vi "gyro_get_statistics.vi"(8 "error in":errorcluster, 11 "all in one package in":T1 {"time informations"."length" format="%<%H:%M:%S%3u>t"; "actigraph settings"."id" format="%02d"; "actigraph settings"."range code" format="%02x"; "actigraph settings"."rate code" format="%02x"}) -> (0 "error out":errorcluster, 3 "all in one package out":T1 {"time informations"."length" format="%<%H:%M:%S%3u>t"; "actigraph settings"."id" format="%02d"; "actigraph settings"."range code" format="%02x"; "actigraph settings"."rate code" format="%02x"})   [LabVIEW 2019]
uses:
  <vilib>/Analysis/NI_AALBase.lvlib
  Controls/gyro_control_memory_structure.ctl
  Controls/gyro_control_measurement_settings.ctl
  Controls/gyro_control_time_informations.ctl
  Controls/gyro_control_measurement_data.ctl
  Controls/gyro_control_all_in_one_package.ctl
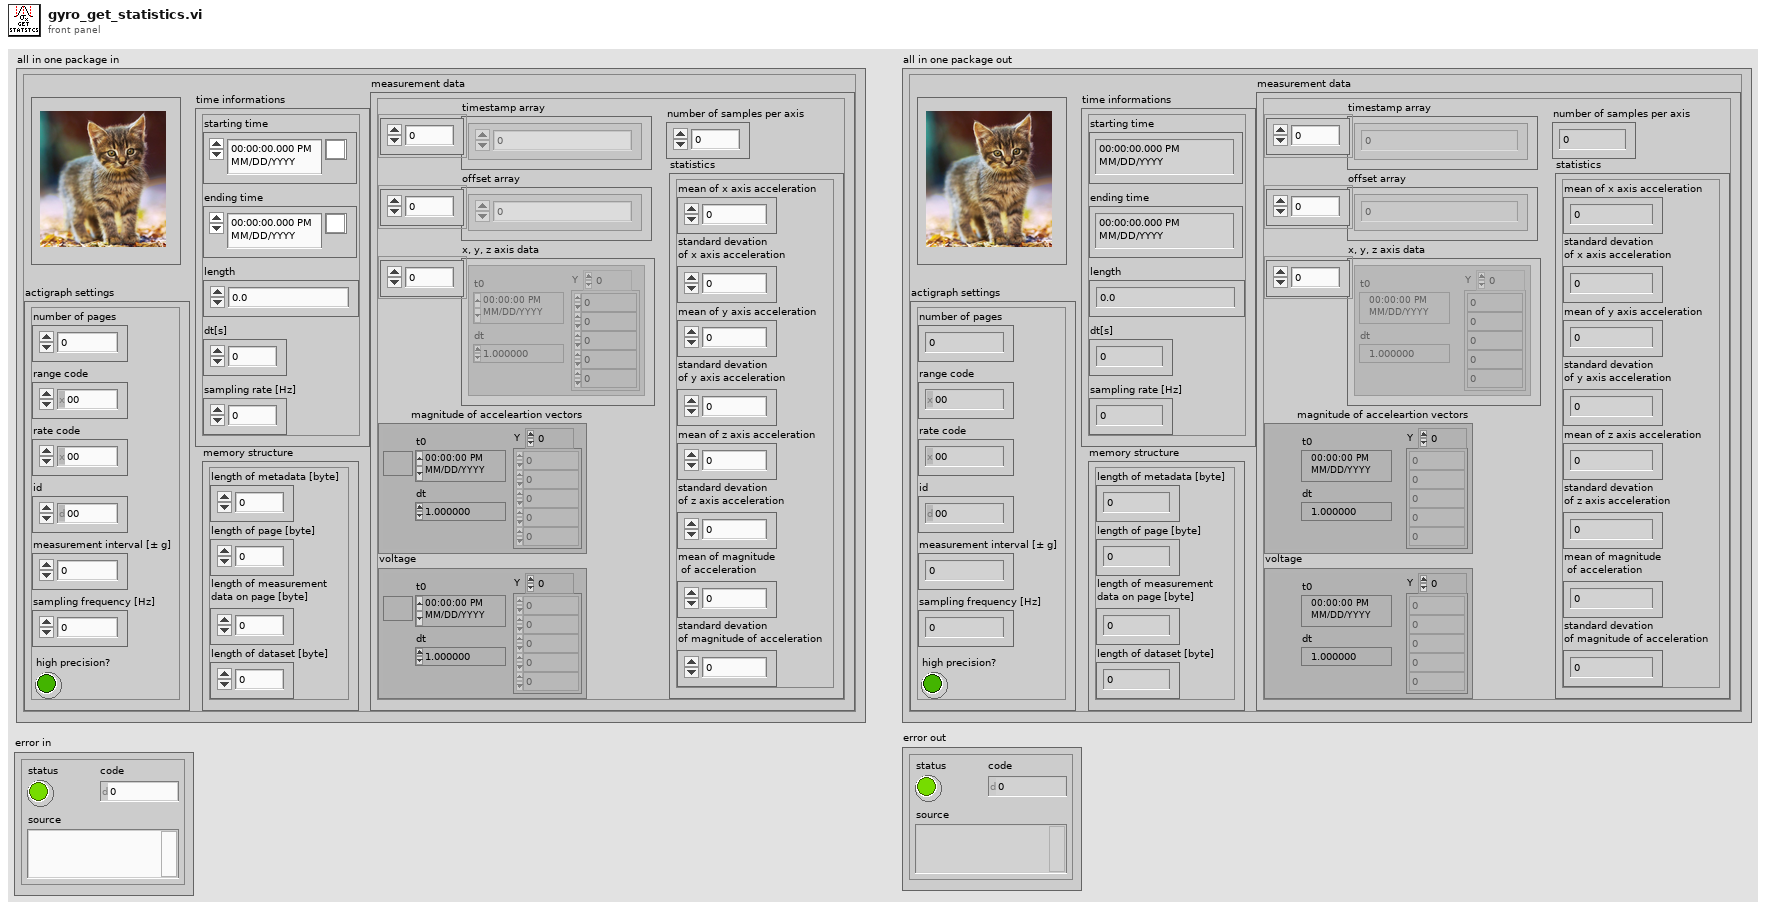
[diagram p1: front panel]
types:
  T1 = typedef "gyro_control_all_in_one_package.ctl" = cluster{"measurement data":T2, "actigraph settings":T3, "memory structure":T4, "time informations":T5}
  T2 = typedef "gyro_control_measurement_data.ctl" = cluster{"number of samples per axis":i32, "timestamp array":dbl[], "offset array":dbl[], "x, y, z axis data":waveform(dbl)[], "magnitude of acceleartion vectors":waveform(dbl), "statistics":cluster{"mean of x axis acceleration":dbl, "standard devation \nof x axis acceleration":dbl, "mean of y axis acceleration":dbl, "standard devation \nof y axis acceleration":dbl, "mean of z axis acceleration":dbl, "standard devation \nof z axis acceleration":dbl, "mean of magnitude\n of acceleration":dbl, "standard devation \nof magnitude of acceleration":dbl}, "voltage":waveform(dbl)}
  T3 = typedef "control_measurement_settings.ctl" = cluster{"sampling frequency [Hz]":dbl, "measurement interval [± g]":i32, "high precision?":bool, "number of pages":i32, "rate code":i32, "range code":i32, "id":i32}
  T4 = typedef "gyro_control_memory_structure.ctl" = cluster{"length of metadata [byte]":i32, "length of page [byte]":i32, "length of measurement \ndata on page [byte]":i32, "length of dataset [byte]":i32}
  T5 = typedef "gyro_control_time_informations.ctl" = cluster{"starting time":timestamp, "ending time":timestamp, "dt[s]":dbl, "sampling rate [Hz]":dbl, "length":dbl}
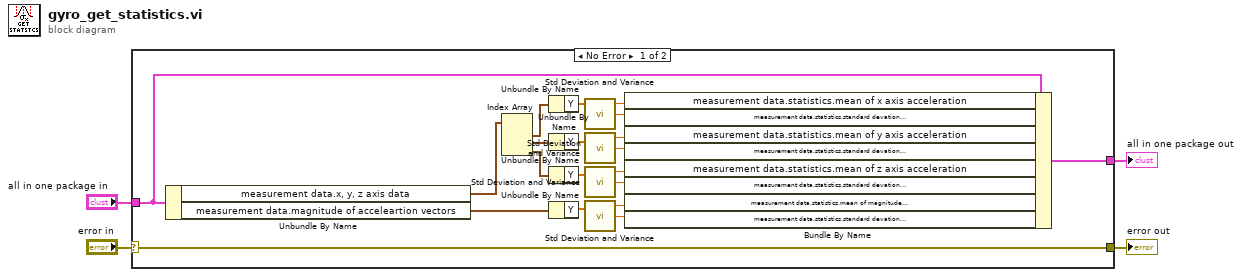
[diagram p0: block diagram]
diagram:
  n1 = case shown="No Error" "error in" {
    selector: "error in" -> [w24 w25]
    tunnel: [w24 w25] -> w3
    tunnel: "all in one package in" -> [w16 w26]
    tunnel: [w15 w26] -> w1
    frame No Error {
      n2 = Unbundle By Name(w16) -> ("measurement data.x, y, z axis data"=w23:waveform(dbl)[], "measurement data.magnitude of acceleartion vectors"=w17:waveform(dbl))
      n3 = Index Array(array=w23) -> (element #1=w22:waveform(dbl), element #2=w21:waveform(dbl), element #3=w20:waveform(dbl))  [unwired: 3 in]
      n4 = Unbundle By Name(w22) -> ("Y"=w19:dbl[])
      n5 = Unbundle By Name(w21) -> ("Y"=w18:dbl[])
      n6 = Unbundle By Name(w20) -> ("Y"=w6:dbl[])
      n7 = Unbundle By Name(w17) -> ("Y"=w5:dbl[])
      n8 = call <vilib>:"Std Deviation and Variance.vi"("X"=w19) -> ("mean"=w14:dbl, "standard deviation"=w13:dbl)  [unwired: 1 in, 1 out]
      n9 = call <vilib>:"Std Deviation and Variance.vi"("X"=w18) -> ("mean"=w12:dbl, "standard deviation"=w11:dbl)  [unwired: 1 in, 1 out]
      n10 = call <vilib>:"Std Deviation and Variance.vi"("X"=w6) -> ("mean"=w10:dbl, "standard deviation"=w9:dbl)  [unwired: 1 in, 1 out]
      n11 = call <vilib>:"Std Deviation and Variance.vi"("X"=w5) -> ("mean"=w8:dbl, "standard deviation"=w7:dbl)  [unwired: 1 in, 1 out]
      n12 = Bundle By Name(cluster=w16, "measurement data.statistics.mean of x axis acceleration"=w14, "measurement data.statistics.standard devation \nof x axis acceleration"=w13, "measurement data.statistics.mean of y axis acceleration"=w12, "measurement data.statistics.standard devation \nof y axis acceleration"=w11, "measurement data.statistics.mean of z axis acceleration"=w10, "measurement data.statistics.standard devation \nof z axis acceleration"=w9, "measurement data.statistics.mean of magnitude\n of acceleration"=w8, "measurement data.statistics.standard devation \nof magnitude of acceleration"=w7) -> (w15:T1)
    }
    frame Error {
    }
  }
  "error out" <- w3
  "all in one package out" <- w1
